vi "CRYTS Read.vi"(10 "Sequence folder path":path, 11 "File Name":string) -> (0 "Sequence Name":string, 1 "Channels":i32, 2 "sequence list":T1, 3 "Header info":T2={"Data type"="Data            ", "Version"=1, "Dimensions"=0}, 4 "Selected Seq Path":path, 5 "status":bool, 6 "Is RecentFile?":bool, 7 "Is Replace?":bool)   [LabVIEW 2013]
uses:
  Control/CRYSequence Cluster.ctl
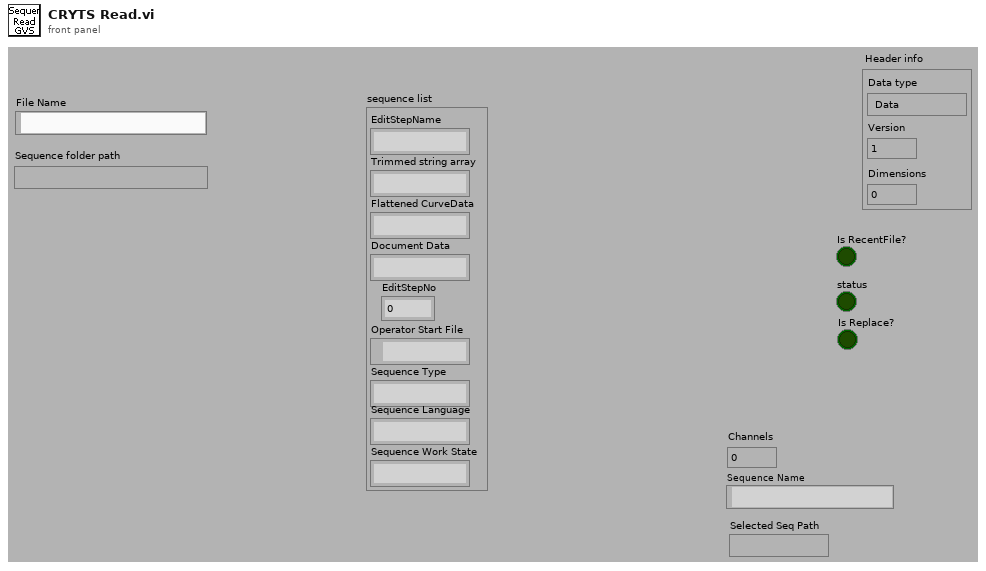
[diagram p1: front panel]
types:
  T1 = typedef "CRYSequence Cluster.ctl" = cluster{"EditStepName":string, "Trimmed string array":string, "Flattened CurveData":string, "Document Data":string, "EditStepNo":u16, "Operator Start File":path, "Sequence Type":string, "Sequence Language":string, "Sequence Work State":string}
  T2 = cluster{"Data type":string, "Version":u16, "Dimensions":u8}
  T3 = cluster{"EditStepName":string, "Trimmed string array":string, "Flattened CurveData":string}
  T4 = cluster{"EditStepName":string, "Trimmed string array":string, "Flattened CurveData":string, "Document Data":string}
  T5 = cluster{"EditStepName":string, "Trimmed string array":string, "Flattened CurveData":string, "Document Data":string, "EditStepNo":u16}
  T6 = cluster{"EditStepName":string, "Trimmed string array":string, "Flattened CurveData":string, "Document Data":string, "EditStepNo":u16, "Operator Start File":path}
  T7 = cluster{"EditStepName":string, "Trimmed string array":string, "Flattened CurveData":string, "Document Data":string, "EditStepNo":u16, "Operator Start File":path, "Sequence Type":string}
  T8 = cluster{"EditStepName":string, "Trimmed string array":string, "Flattened CurveData":string, "Document Data":string, "EditStepNo":u16, "Operator Start File":path, "Sequence Type":string, "Sequence Language":string}
  T9 = cluster{"unsigned byte array[0]":u8, "unsigned byte array[1]":u8, "unsigned byte array[2]":u8}
  T10 = cluster{"EditStepName":string, "Trimmed string array":string, "Flattened CurveData":string}[]
  T11 = cluster{"EditStepName":string, "Trimmed string array":string, "Flattened CurveData":string, "Document Data":string}[]
  T12 = cluster{"EditStepName":string, "Trimmed string array":string, "Flattened CurveData":string, "Document Data":string, "EditStepNo":u16}[]
  T13 = cluster{"EditStepName":string, "Trimmed string array":string, "Flattened CurveData":string, "Document Data":string, "EditStepNo":u16, "Operator Start File":path}[]
  T14 = cluster{"EditStepName":string, "Trimmed string array":string, "Flattened CurveData":string, "Document Data":string, "EditStepNo":u16, "Operator Start File":path, "Sequence Type":string}[]
  T15 = cluster{"EditStepName":string, "Trimmed string array":string, "Flattened CurveData":string, "Document Data":string, "EditStepNo":u16, "Operator Start File":path, "Sequence Type":string, "Sequence Language":string}[]
  T16 = cluster{string, u16, "unsigned byte array[2]":u8}
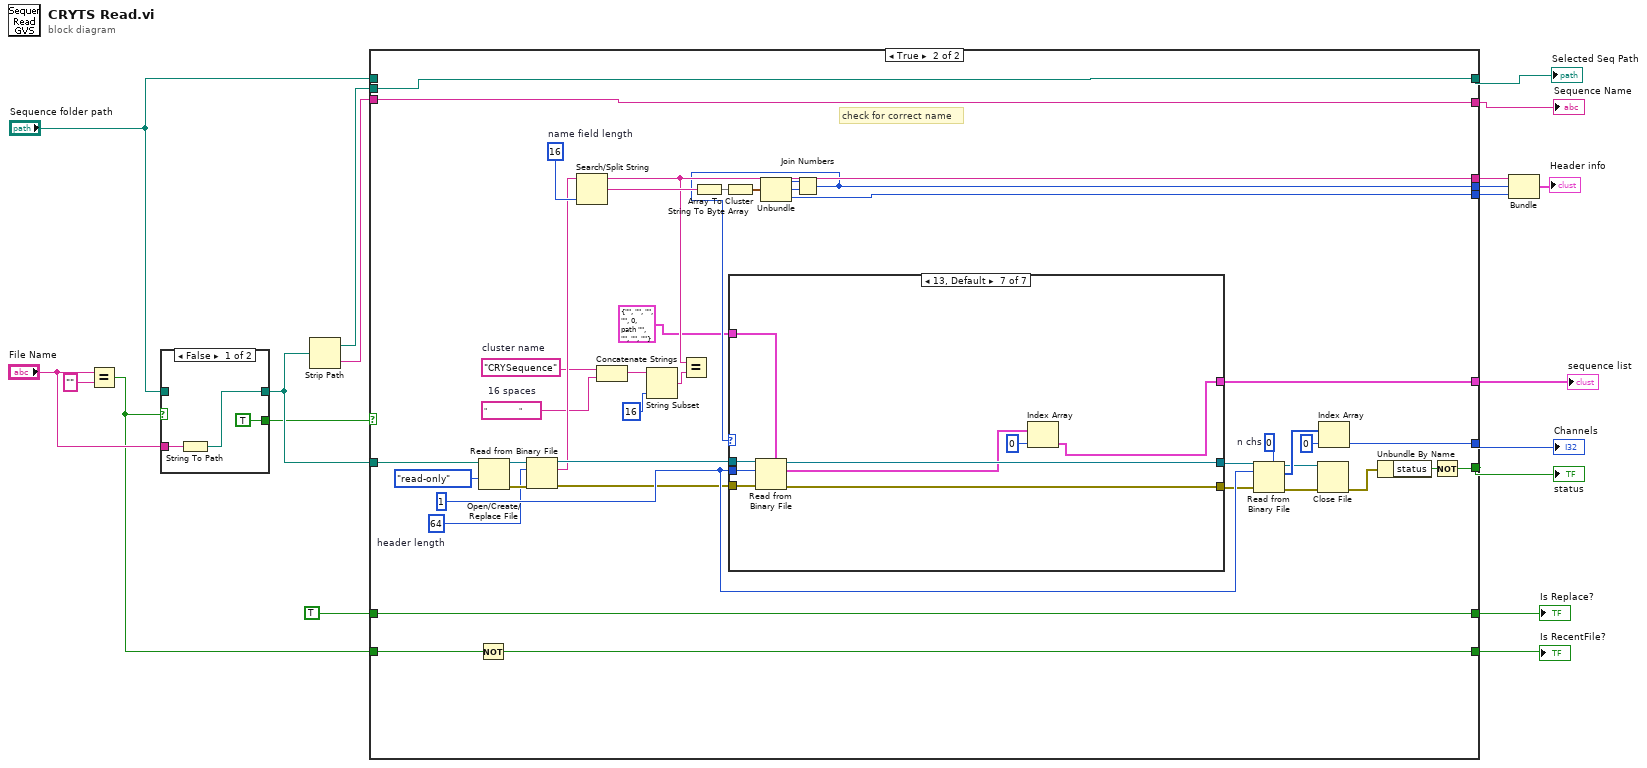
[diagram p0: block diagram]
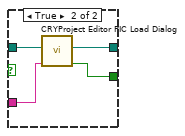
[diagram p2: hidden frame]
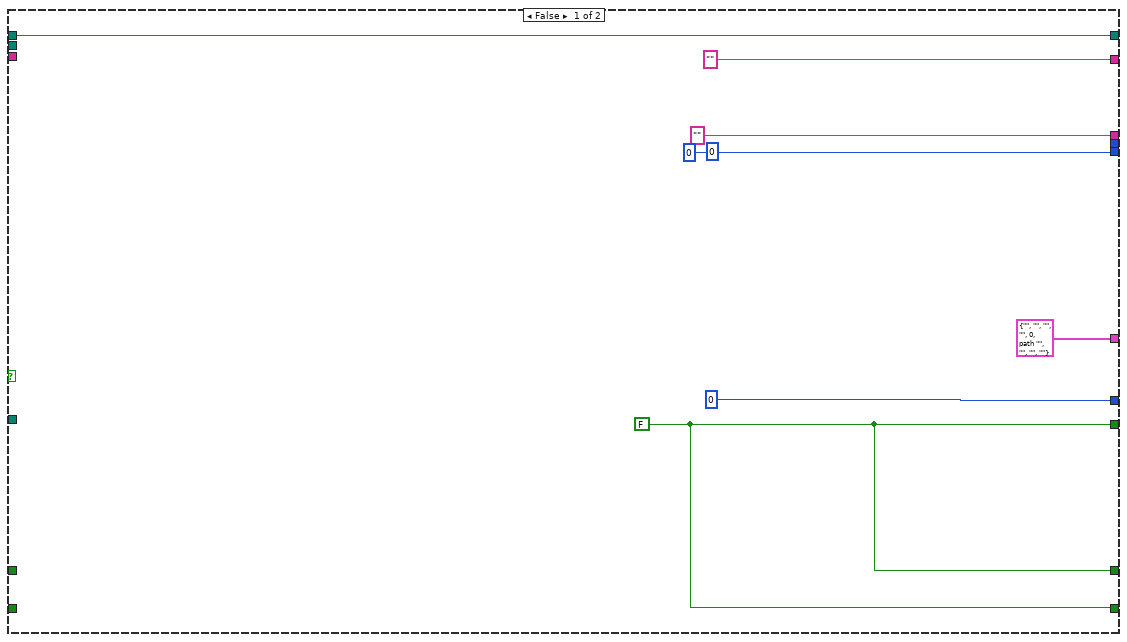
[diagram p3: hidden frame]
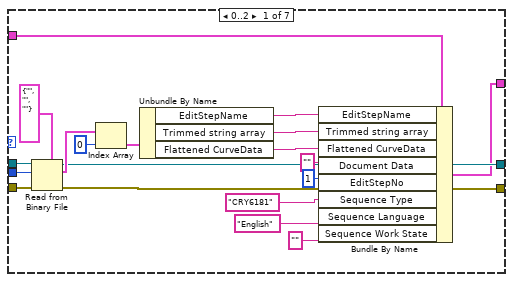
[diagram p4: hidden frame]
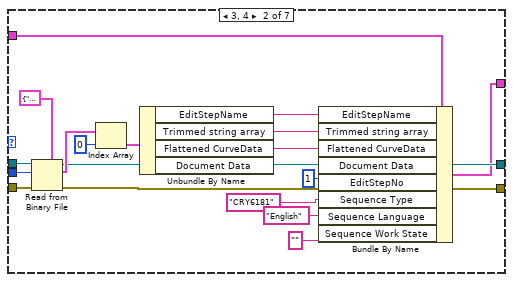
[diagram p5: hidden frame]
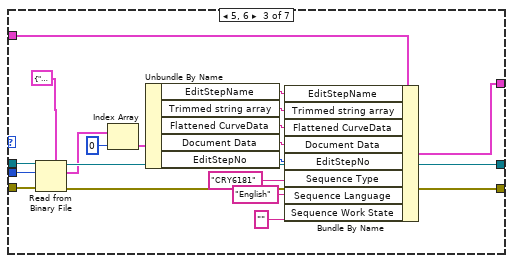
[diagram p6: hidden frame]
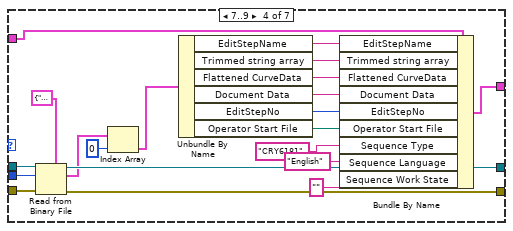
[diagram p7: hidden frame]
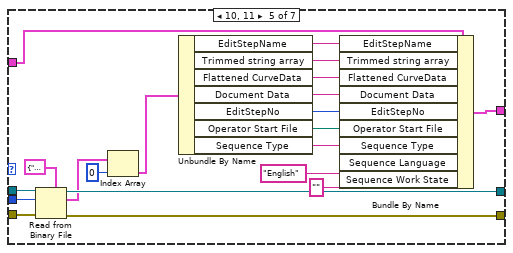
[diagram p8: hidden frame]
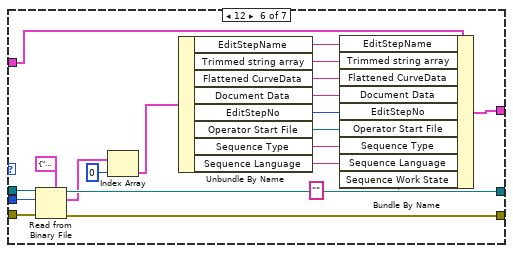
[diagram p9: hidden frame]
diagram:
  n1 = Equal?(x="File Name", y="") -> (x = y?=w15:bool)
  n2 = case shown="False" w15 {
    tunnel: [w21 w25] -> w7
    tunnel: [TRUE w24] -> w3
    tunnel: "Sequence folder path" -> [_ w27]
    tunnel: "File Name" -> [w22 w26]
    frame False {
      n3 = String To Path(string=w22) -> (path=w21:path)
    }
    frame True {
      n4 = call "CRYProject Editor PIC Load Dialog.vi"("File Name"=w26, "Sequence folder path"=w27) -> ("bResult"=w24:bool, "pPathFull"=w25:path)  [unwired: 8 in]
    }
  }
  n5 = Strip Path(path=w7) -> (stripped path=w6:path, name=w5:string)
  n6 = case shown="True" w3 {
    tunnel: w7 -> [_ w68]
    tunnel: [w29 w66] -> w20
    tunnel: ["" ("name") w39] -> w19
    tunnel: [T1 {"EditStepName"="", "Trimmed string array"="", "Flattened CurveData"="", "Document Data"="", "EditStepNo"=0, "Operator Start File"=path "", "Sequence Type"="", "Sequence Language"="", "Sequence Work State"=""} ("output cluster") w37] -> w1
    tunnel: [0 ("n chs") w69] -> w18
    tunnel: w15 -> [_ w67]
    tunnel: [w33 w40] -> w13
    tunnel: "Sequence folder path" -> [w33 _]
    tunnel: [w29 w65] -> w12
    tunnel: [u16 0 w41] -> w10
    tunnel: [u8 0 ("unsigned byte array[2]") w57] -> w9
    tunnel: ["" w51] -> w8
    tunnel: w6 -> [_ w40]
    tunnel: w5 -> [_ w39]
    tunnel: TRUE -> [_ w38]
    tunnel: [w29 w38] -> w4
    frame False {
      w29 = FALSE
    }
    frame True {
      w50 = 0  # n chs
      w56 = "                "  # 16 spaces
      w53 = "CRYSequence"  # cluster name
      w64 = 16  # name field length
      w71 = 64  # header length
      w76 = 1
      # "check for correct name"
      n7 = Not(x=w67) -> (.not. x?=w65:bool)
      n8 = Open/Create/Replace File(file path (use dialog)=w68, access (0:read/write)=enum16{"read/write", "read-only", "write-only"}."read-only") -> (refnum out=w74:refnum<file>, error out=w75:errorcluster)  [unwired: 1 in, 4 out]
      n9 = Read from Binary File(8:w75, 10:w71, 11:w74) -> (0:w73:errorcluster, 2:w63:string, 3:w72:refnum<file>)  [unwired: 4 out]
      n10 = Search/Split String(string=w63, offset (0)=w64) -> (substring before match=w51:string, match + rest of string=w58:string)  [unwired: 2 out]
      n11 = Concatenate Strings(w53, w56) -> (w54:string)
      n12 = String Subset(string=w54, length (rest)=16 ("length (rest)")) -> (substring=w52:string)  [unwired: 1 out]
      n13 = Equal?(x=w51, y=w52) -> ()  [unwired: 1 out]
      n14 = String To Byte Array(string=w58) -> (unsigned byte array=w59:u8[])
      n15 = Array To Cluster(array=w59) -> (cluster=w60:T9)
      n16 = Unbundle(w60) -> ("unsigned byte array[0]"=w61:u8, "unsigned byte array[1]"=w62:u8, "unsigned byte array[2]"=w57:u8)
      n17 = Join Numbers(hi=w61, lo=w62) -> ((hi.lo)=w41:u16)
      n18 = case shown="13, Default" w41 {
        tunnel: w76 -> [w91 w111 w133 w153 w173 w193 w202]
        tunnel: w73 -> [w90 w110 w132 w152 w172 w192 w201]
        tunnel: w72 -> [w92 w112 w131 w151 w171 w191 w200]
        tunnel: [w79 w103 w119 w137 w158 w178 w195] -> w37
        tunnel: [w88 w108 w130 w150 w170 w190 w199] -> w49
        tunnel: [w89 w109 w129 w149 w169 w189 w198] -> w48
        tunnel: T1 {"EditStepName"="", "Trimmed string array"="", "Flattened CurveData"="", "Document Data"="", "EditStepNo"=0, "Operator Start File"=path "", "Sequence Type"="", "Sequence Language"="", "Sequence Work State"=""} ("output cluster") -> [w81 w99 w118 w138 w159 w179 w194]
        frame 0..2 {
          n19 = Read from Binary File(5:T3 {"EditStepName"="", "Trimmed string array"="", "Flattened CurveData"=""} ("sequence list"), 8:w90, 10:w91, 11:w92) -> (0:w89:errorcluster, 2:w95:T10, 3:w88:refnum<file>)  [unwired: 3 out]
          n20 = Index Array(array=w95, index=0) -> (element=w87:T3)
          n21 = Unbundle By Name(w87) -> ("EditStepName"=w86:string, "Trimmed string array"=w85:string, "Flattened CurveData"=w84:string)
          n22 = Bundle By Name(cluster=w81, "EditStepName"=w86, "Trimmed string array"=w85, "Flattened CurveData"=w84, "Document Data"="", "EditStepNo"=u16 1, "Sequence Type"="CRY6181" ("Section"), "Sequence Language"="English", "Sequence Work State"="") -> (w79:T1)
        }
        frame 3, 4 {
          n23 = Read from Binary File(5:T4 {"EditStepName"="", "Trimmed string array"="", "Flattened CurveData"="", "Document Data"=""} ("sequence list"), 8:w110, 10:w111, 11:w112) -> (0:w109:errorcluster, 2:w114:T11, 3:w108:refnum<file>)  [unwired: 3 out]
          n24 = Index Array(array=w114, index=0) -> (element=w107:T4)
          n25 = Unbundle By Name(w107) -> ("EditStepName"=w106:string, "Trimmed string array"=w105:string, "Flattened CurveData"=w104:string, "Document Data"=w100:string)
          n26 = Bundle By Name(cluster=w99, "EditStepName"=w106, "Trimmed string array"=w105, "Flattened CurveData"=w104, "Document Data"=w100, "EditStepNo"=u16 1, "Sequence Type"="CRY6181" ("Section"), "Sequence Language"="English", "Sequence Work State"="") -> (w103:T1)
        }
        frame 5, 6 {
          n27 = Read from Binary File(5:T5 {"EditStepName"="", "Trimmed string array"="", "Flattened CurveData"="", "Document Data"="", "EditStepNo"=0} ("sequence list"), 8:w132, 10:w133, 11:w131) -> (0:w129:errorcluster, 2:w128:T12, 3:w130:refnum<file>)  [unwired: 3 out]
          n28 = Index Array(array=w128, index=0) -> (element=w125:T5)
          n29 = Unbundle By Name(w125) -> ("EditStepName"=w120:string, "Trimmed string array"=w121:string, "Flattened CurveData"=w122:string, "Document Data"=w123:string, "EditStepNo"=w124:u16)
          n30 = Bundle By Name(cluster=w118, "EditStepName"=w120, "Trimmed string array"=w121, "Flattened CurveData"=w122, "Document Data"=w123, "EditStepNo"=w124, "Sequence Type"="CRY6181" ("Section"), "Sequence Language"="English", "Sequence Work State"="") -> (w119:T1)
        }
        frame 7..9 {
          n31 = Read from Binary File(5:T6 {"EditStepName"="", "Trimmed string array"="", "Flattened CurveData"="", "Document Data"="", "EditStepNo"=0, "Operator Start File"=path ""} ("sequence list"), 8:w152, 10:w153, 11:w151) -> (0:w149:errorcluster, 2:w148:T13, 3:w150:refnum<file>)  [unwired: 3 out]
          n32 = Index Array(array=w148, index=0) -> (element=w145:T6)
          n33 = Unbundle By Name(w145) -> ("EditStepName"=w144:string, "Trimmed string array"=w143:string, "Flattened CurveData"=w142:string, "Document Data"=w141:string, "EditStepNo"=w140:u16, "Operator Start File"=w139:path)
          n34 = Bundle By Name(cluster=w138, "EditStepName"=w144, "Trimmed string array"=w143, "Flattened CurveData"=w142, "Document Data"=w141, "EditStepNo"=w140, "Operator Start File"=w139, "Sequence Type"="CRY6181" ("Section"), "Sequence Language"="English", "Sequence Work State"="") -> (w137:T1)
        }
        frame 10, 11 {
          n35 = Read from Binary File(5:T7 {"EditStepName"="", "Trimmed string array"="", "Flattened CurveData"="", "Document Data"="", "EditStepNo"=0, "Operator Start File"=path "", "Sequence Type"=""} ("output cluster"), 8:w172, 10:w173, 11:w171) -> (0:w169:errorcluster, 2:w168:T14, 3:w170:refnum<file>)  [unwired: 3 out]
          n36 = Index Array(array=w168, index=0) -> (element=w166:T7)
          n37 = Unbundle By Name(w166) -> ("EditStepName"=w165:string, "Trimmed string array"=w164:string, "Flattened CurveData"=w163:string, "Document Data"=w162:string, "EditStepNo"=w161:u16, "Operator Start File"=w160:path, "Sequence Type"=w156:string)
          n38 = Bundle By Name(cluster=w159, "EditStepName"=w165, "Trimmed string array"=w164, "Flattened CurveData"=w163, "Document Data"=w162, "EditStepNo"=w161, "Operator Start File"=w160, "Sequence Type"=w156, "Sequence Language"="English", "Sequence Work State"="") -> (w158:T1)
        }
        frame 12 {
          n39 = Read from Binary File(5:T8 {"EditStepName"="", "Trimmed string array"="", "Flattened CurveData"="", "Document Data"="", "EditStepNo"=0, "Operator Start File"=path "", "Sequence Type"="", "Sequence Language"=""} ("output cluster"), 8:w192, 10:w193, 11:w191) -> (0:w189:errorcluster, 2:w188:T15, 3:w190:refnum<file>)  [unwired: 3 out]
          n40 = Index Array(array=w188, index=0) -> (element=w186:T8)
          n41 = Unbundle By Name(w186) -> ("EditStepName"=w185:string, "Trimmed string array"=w184:string, "Flattened CurveData"=w183:string, "Document Data"=w182:string, "EditStepNo"=w181:u16, "Operator Start File"=w180:path, "Sequence Type"=w177:string, "Sequence Language"=w175:string)
          n42 = Bundle By Name(cluster=w179, "EditStepName"=w185, "Trimmed string array"=w184, "Flattened CurveData"=w183, "Document Data"=w182, "EditStepNo"=w181, "Operator Start File"=w180, "Sequence Type"=w177, "Sequence Language"=w175, "Sequence Work State"="") -> (w178:T1)
        }
        frame 13, Default {
          n43 = Read from Binary File(5:w194, 8:w201, 10:w202, 11:w200) -> (0:w198:errorcluster, 2:w197:T1[], 3:w199:refnum<file>)  [unwired: 3 out]
          n44 = Index Array(array=w197, index=0) -> (element=w195:T1)
        }
      }
      n45 = Read from Binary File(5:w50, 8:w48, 10:w76, 11:w49) -> (0:w42:errorcluster, 2:w47:i32[], 3:w43:refnum<file>)  [unwired: 3 out]
      n46 = Close File(refnum=w43, error in=w42) -> (error out=w44:errorcluster)  [unwired: 1 out]
      n47 = Index Array(array=w47, index=0) -> (element=w69:i32)
      n48 = Unbundle By Name(w44) -> ("status"=w45:bool)
      n49 = Not(x=w45) -> (.not. x?=w66:bool)
    }
  }
  "status" <- w20
  "Sequence Name" <- w19
  "Channels" <- w18
  "Selected Seq Path" <- w13
  "Is RecentFile?" <- w12
  "Is Replace?" <- w4
  "sequence list" <- w1
  n50 = Bundle(w8, w10, "unsigned byte array[2]"=w9) -> (→"Header info":T16)  [unwired: 1 out]
